vi "NI9205_SUB-VI_Mean.vi"(11 "Y":dbl[](array[numeric])) -> (3 "Numeric":dbl)   [LabVIEW 2020]
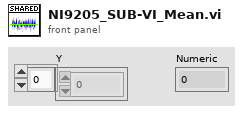
[diagram p1: front panel]
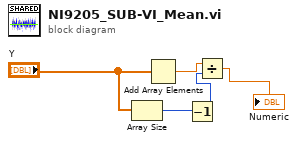
[diagram p0: block diagram]
diagram:
  n1 = Array Size(array="Y") -> (size(s)=w1:i32)
  n2 = Add Array Elements(numeric array="Y") -> (sum=w2:dbl)
  n3 = Decrement(x=w1) -> (x-1=w3:i32)
  n4 = Divide(x=w2, y=w3) -> (x/y=→"Numeric":dbl)
